vi "Get Enabled Routing Channels.vi"(8 "error in (no error)":errorcluster, 11 "Routing Channels Ref in":T1 format="%.0x") -> (0 "error out":errorcluster, 2 "Routing Channel Refs":T1[](array[typedef]) format="%.0x", 3 "Routing Channels Ref out":T1 format="%.0x")   [LabVIEW 2020, in "Routing and Faulting System Explorer.lvlib"]
uses:
  Routing and Faulting System Explorer.lvlib
  <vilib>/NI VeriStand/Custom Device API/Custom Device Item Ref.ctl
  NationalInstruments.VeriStand.SystemDefinitionAPI
  Shared/Constants.vi
  Shared/Routing and Faulting Shared.lvlib
  <vilib>/NI VeriStand/Custom Device API/Custom Device API.lvlib
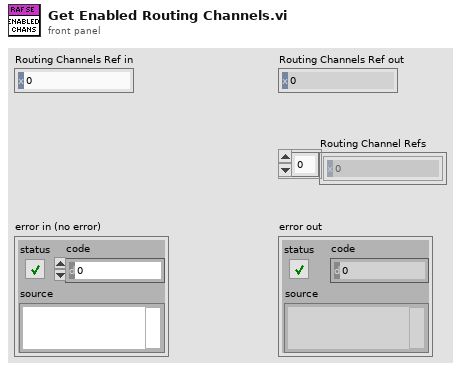
[diagram p1: front panel]
types:
  T1 = typedef "Custom Device API.lvlib/Custom Device Item Ref.ctl" = u64
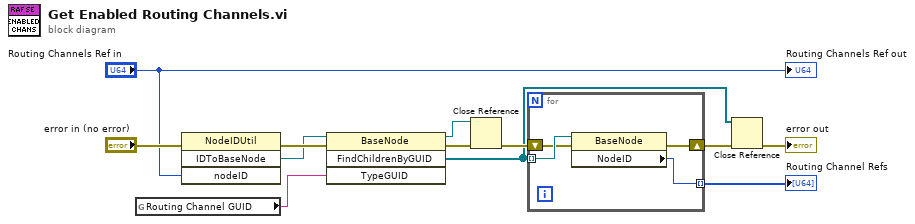
[diagram p0: block diagram]
diagram:
  n1 = global read "Constants.vi" "Routing Channel GUID"() -> (w8:string)
  n2 = invoke class="NodeIDUtil" method="IDToBaseNode"(error in="error in (no error)", "nodeID"="Routing Channels Ref in") -> (error out=w10:errorcluster, "IDToBaseNode"=w9:refnum<k24>)  [unwired: 2 in, 2 out]
  n3 = invoke class="BaseNode" method="FindChildrenByGUID"(reference=w9, error in=w10, "TypeGUID"=w8) -> (reference out=w6:refnum<k24>, error out=w7:errorcluster, "FindChildrenByGUID"=w1:refnum<k24>[])  [unwired: 1 in, 1 out]
  n4 = Close Reference(reference=w6, error in (no error)=w7) -> (error out=w5:errorcluster)
  n5 = for {
    tunnel: w1 -> [w16] mode=indexing
    shift-right: [w14] -> w4
    shift-left: w5 -> [w15]
    tunnel: [w13] -> w3 mode=indexing
    n6 = property class="BaseNode"(reference=w16, error in=w15) -> (error out=w14:errorcluster, "NodeID"=w13:u64)  [unwired: 1 out]
  }
  "Routing Channel Refs" <- w3
  n7 = Close Reference(reference=w1, error in (no error)=w4) -> (error out=→"error out":errorcluster)
  "Routing Channels Ref out" <- "Routing Channels Ref in"
